vi "re_VI.abort_lua.vi"(5 "LuaVIEW reference":T1) -> (15 "error out":errorcluster)   [LabVIEW 2012]
doc: "Aborts a VI. This method maps to the LabVIEW abort VI method. Beware that the VI is not given a chance to do any cleanup work. When this is a problem, consider using a plug-in.\n\nThis function is reentrant because the abort VI method can take a while and might even get stuck without timing out in certain pathological cases, particularly when the VI being aborted has called a DLL function that fails to return.\nParameters:\nobj:self, object of VI to abort.\nErrors:\nNot a VI object.\nDead VI object.\nCould not abort VI."
uses:
  typedefs/t_LuaVIEW Reference.ctl
  subvis/private/LuaVIEW Pull (object).vi
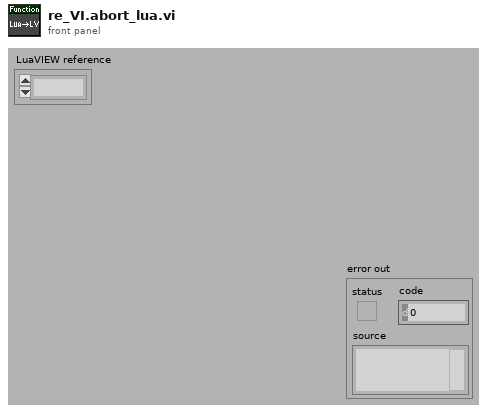
[diagram p1: front panel]
types:
  T1 = typedef "t_LuaVIEW Reference.ctl" = refnum<k1>
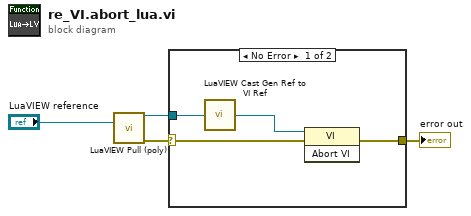
[diagram p0: block diagram]
diagram:
  n1 = call-poly "LuaVIEW Pull (poly).vi"("LuaVIEW reference in"="LuaVIEW reference") -> ("object refnum"=w2:refnum<vi>, "error out"=w1:errorcluster)  [unwired: 11 in, 2 out]
  n2 = case shown="No Error" w1 {
    selector: w1 -> [w8 w9]
    tunnel: [w6 w9] -> w3
    tunnel: w2 -> [w5 _]
    frame No Error {
      n3 = call "LuaVIEW Cast Gen Ref to VI Ref.vi"("refnum in"=w5) -> ("refnum out"=w7:refnum<vi>)  [unwired: 14 in]
      n4 = invoke class="VI" method="Abort VI"(reference=w7, error in=w8) -> (error out=w6:errorcluster)  [unwired: 1 in, 2 out]
    }
    frame Error {
    }
  }
  "error out" <- w3
